vi "Get XSDVersion.vi"(8 "error in":errorcluster, 11 "XML Node":refnum<k20>) -> (0 "error out":errorcluster, 2 "XSDVersion":T1, 3 "XML Node out":refnum<k20>)   [LabVIEW 2024, in "Config File Parser.lvlib" / "Custom Device Config.lvclass"]
uses:
  Custom Device Config.lvclass
  XSDVersion.ctl
  <vilib>/xml/Close Reference(Node).vi
  Custom Device Config.lvclass/Custom Device Config.ctl
  <resource>/objmgr/DOMUserDefRef.rc
  <vilib>/xml/NI_XML.lvlib
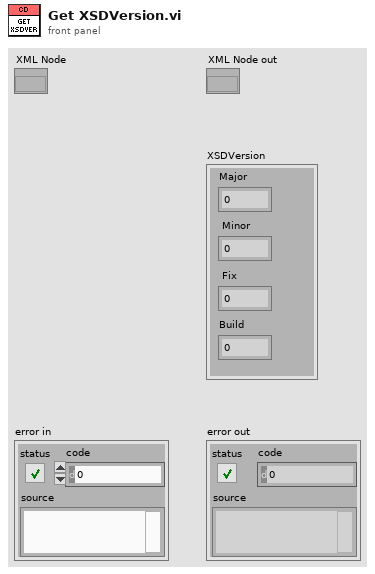
[diagram p1: front panel]
types:
  T1 = typedef "Config File Parser.lvlib/Custom Device Config.lvclass/XSDVersion.ctl" = cluster{"Major":u32, " Minor":u32, " Fix":u32, "Build":u32}
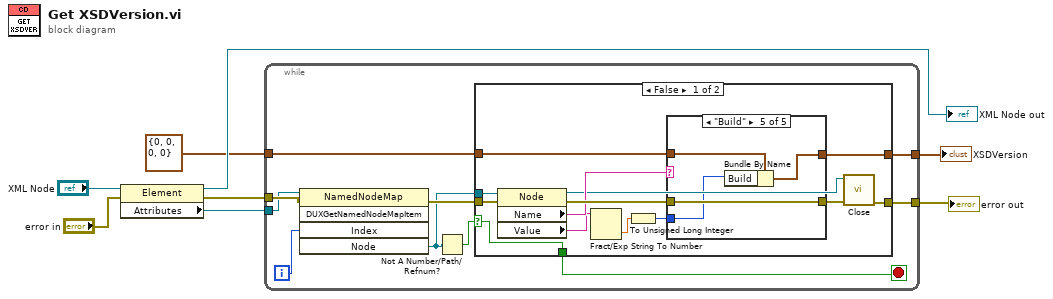
[diagram p0: block diagram]
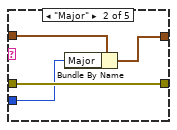
[diagram p3: hidden frame]
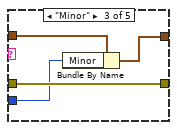
[diagram p4: hidden frame]
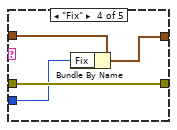
[diagram p5: hidden frame]
diagram:
  n1 = property on="Property Node" class="Element"(reference="XML Node", error in="error in") -> (reference out=→"XML Node out":refnum<k20>, error out=w8:errorcluster, "Attributes"=w4:refnum<k20>)
  n2 = while {
    tunnel: w4 -> [w15]
    tunnel: T1 {"Major"=0, " Minor"=0, " Fix"=0, "Build"=0} ("XSDVersion") -> [w14]
    tunnel: [w13] -> w1
    tunnel: w8 -> [w17]
    tunnel: [w16] -> w6
    i -> [w10]
    stop <- w11 stop-if-true
    n3 = invoke on="Invoke Node" class="NamedNodeMap" method="DUXGetNamedNodeMapItem"(reference=w15, error in=w17, "Index"=w10) -> (error out=w18:errorcluster, "Node"=w9:refnum<k20>)  [unwired: 2 in, 3 out]
    n4 = Not A Number/Path/Refnum?(number/path/refnum=w9) -> (NaN/Path/Refnum?=w12:bool)
    n5 = case shown="False" w12 {
      selector: w12 -> [w23 w51]
      tunnel: w18 -> [w31 w52]
      tunnel: [w28 w52] -> w16
      tunnel: [w23 w51] -> w11
      tunnel: [w27 w50] -> w13
      tunnel: w14 -> [w25 w50]
      tunnel: w9 -> [w22 _]
      frame False {
        n6 = property on="Property Node" class="Node"(reference=w22, error in=w31) -> (reference out=w24:refnum<k20>, error out=w30:errorcluster, "Name"=w26:string, "Value"=w20:string)
        n7 = Fract/Exp String To Number(string=w20) -> (number=w21:dbl)  [unwired: 3 in, 1 out]
        n8 = To Unsigned Long Integer(number=w21) -> (unsigned 32bit integer=w19:u32)
        n9 = case shown="\"Build\"" w26 {
          tunnel: [w32 w36 w40 w44 w48] -> w27
          tunnel: w30 -> [w33 w37 w41 w45 w49]
          tunnel: [w33 w37 w41 w45 w49] -> w29
          tunnel: w25 -> [w32 w35 w39 w43 w47]
          tunnel: w19 -> [_ w34 w38 w42 w46]
          frame "-1", Default {
          }
          frame "Major" {
            n10 = Bundle By Name(cluster=w35, "Major"=w34) -> (w36:T1)
          }
          frame "Minor" {
            n11 = Bundle By Name(cluster=w39, "Minor"=w38) -> (w40:T1)
          }
          frame "Fix" {
            n12 = Bundle By Name(cluster=w43, "Fix"=w42) -> (w44:T1)
          }
          frame "Build" {
            n13 = Bundle By Name(cluster=w47, "Build"=w46) -> (w48:T1)
          }
        }
        n14 = call-poly <vilib>:"Close.vi"("error in (no error)"=w29, "node"=w24) -> ("error out"=w28:errorcluster)  [unwired: 7 in]
      }
      frame True {
      }
    }
  }
  "error out" <- w6
  "XSDVersion" <- w1
